vi "XIPIN_CANFD_1_0.vi"   [LabVIEW 2017]
doc: "The Xilinx CANFD core solution is a full featured yet compact core. It conforms to the ISO 11898-1:2015, CAN 2.0A and CAN 2.0 B Standards. Bits rates greater than 4 Mbps are supported. The full version of the CANFD core can be purchased and downloaded from the Xilinx IP Center: http://www.xilinx.com/ipcenter/. Note that CAN FD IP user needs to buy Protocol License from Robert Bosch to before selling a device containing the CAN FD IP core\n------------------------------------\n<b>Need License</b> : Yes\n<b>Interface</b> : AXI4"
uses:
  <vilib>/rvi/XilinxIP/XIPIN_XNode/niFpgaXIPIN.xnode
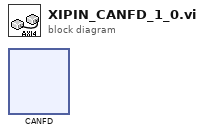
[diagram p0: block diagram]
diagram:
  n1 = xnode ("CANFD")() -> ()
